vi "Loop_SEN.vi"() -> ()   [LabVIEW 2017, in "TemplateSensor.lvlib"]
uses:
  TemplateSensor.lvlib
  _SHARE ALL/Global Share All/Global_STOP.vi
  Global_CMD.vi
  Global_SEN Write_Data.vi
panel:
  out "Output Data":dbl
  out "Input Data":bool
  out "Cycle Time (S)":dbl format="%.3g"
  in  "Target Time(ms)":u32=50
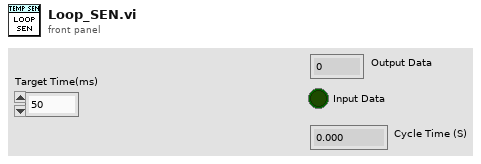
[diagram p1: front panel]
types:
  T1 = cluster{"Sensor Ref Data":cluster{i32}, " Sensor Output":dbl, "Sesnor Input":bool, "Target Time(ms)":u32, "Current Time":timestamp, "Previous Time":timestamp, "Cycle Time (S)":dbl}
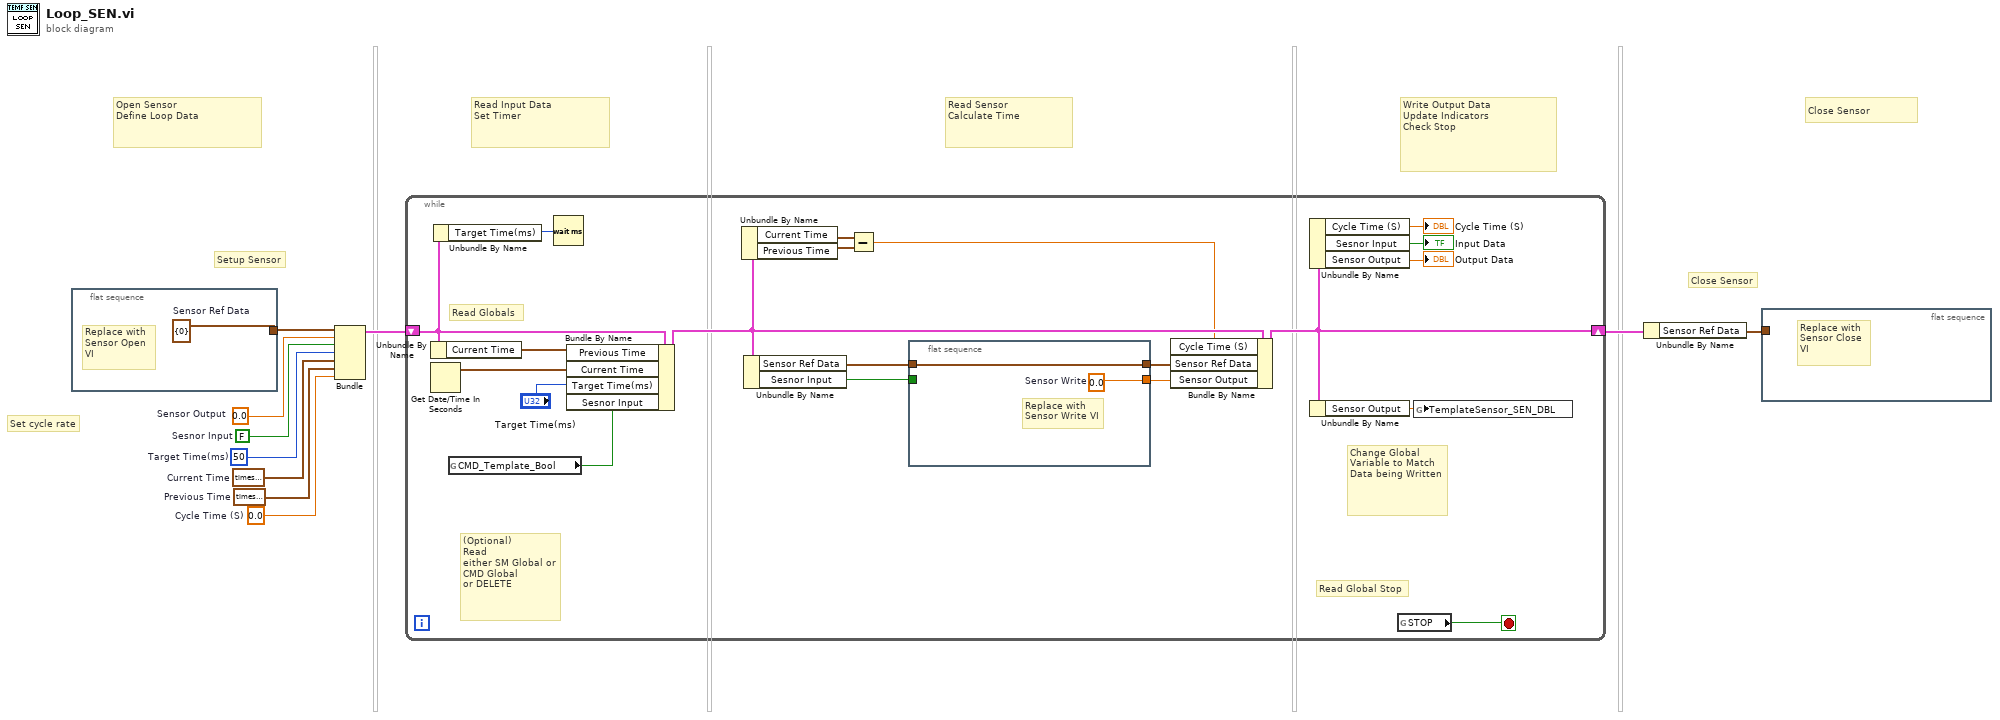
[diagram p0: block diagram]
diagram:
  w1 = 0.0  # Cycle Time (S)
  w10 = timestamp(0 s since 1904-01-01)  # Previous Time
  w9 = timestamp(0 s since 1904-01-01)  # Current Time
  w8 = u32 50  # Target Time(ms)
  w6 = FALSE  # Sesnor Input
  w4 = 0.0  # Sensor Output
  # "Close Sensor"
  # "Write Output Data\nUpdate Indicators\nCheck Stop"
  # "Read Sensor\nCalculate Time"
  # "Read Input Data\nSet Timer"
  # "Open Sensor\nDefine Loop Data"
  # "Set cycle rate"
  # "Close Sensor"
  # "Setup Sensor"
  n1 = flat-sequence {
    tunnel: [w11] -> w3
    frame #0 {
      w11 = cluster{i32} {0}  # Sensor Ref Data
      # "Replace with \nSensor Open\nVI"
    }
  }
  n2 = Bundle("Sensor Ref Data"=w3, "Sensor Output"=w4, "Sesnor Input"=w6, "Target Time(ms)"=w8, "Current Time"=w9, "Previous Time"=w10, "Cycle Time (S)"=w1) -> (w5:T1)  [unwired: 1 in]
  n3 = while {
    shift-right: [w17] -> w2
    shift-left: w5 -> [w19]
    stop <- w31 stop-if-true
    # "Change Global\nVariable to Match\nData being Written"
    # "(Optional)\nRead\neither SM Global or CMD Global\nor DELETE"
    # "Read Globals"
    # "Read Global Stop"
    n4 = Unbundle By Name(w19) -> ("Current Time"=w24:timestamp)
    n5 = Get Date/Time In Seconds() -> (seconds since 1Jan1904=w25:timestamp)
    n6 = Unbundle By Name(w19) -> ("Target Time(ms)"=w18:u32)
    n7 = global read "Global_CMD.vi" "CMD_Template_Bool"() -> (w12:bool)
    n8 = Wait (ms)(milliseconds to wait=w18) -> ()  [unwired: 1 out]
    n9 = Bundle By Name(cluster=w19, "Previous Time"=w24, "Current Time"=w25, "Target Time(ms)"="Target Time(ms)", "Sesnor Input"=w12) -> (w20:T1)
    n10 = Unbundle By Name(w20) -> ("Current Time"=w23:timestamp, "Previous Time"=w22:timestamp)
    n11 = Unbundle By Name(w20) -> ("Sensor Ref Data"=w30:cluster{i32}, "Sesnor Input"=w27:bool)
    n12 = Subtract(x=w23, y=w22) -> (x-y=w13:dbl)
    n13 = flat-sequence {
      tunnel: w30 -> [w33]
      tunnel: [w33] -> w29
      tunnel: [w32] -> w26
      tunnel: w27 -> [_]
      frame #0 {
        w32 = 0.0  # Sensor Write
        # "Replace with\nSensor Write VI"
      }
    }
    n14 = Bundle By Name(cluster=w20, "Cycle Time (S)"=w13, "Sensor Ref Data"=w29, "Sensor Output"=w26) -> (w17:T1)
    n15 = Unbundle By Name(w17) -> ("Cycle Time (S)"=→"Cycle Time (S)":dbl, "Sesnor Input"=→"Input Data":bool, "Sensor Output"=→"Output Data":dbl)
    n16 = Unbundle By Name(w17) -> ("Sensor Output"=w28:dbl)
    n17 = global read "Global_STOP.vi" "STOP"() -> (w31:bool)
    n18 = global write "Global_SEN Write_Data.vi" "TemplateSensor_SEN_DBL"(w28) -> ()
  }
  n19 = Unbundle By Name(w2) -> ("Sensor Ref Data"=w7:cluster{i32})
  n20 = flat-sequence {
    tunnel: w7 -> [_]
    frame #0 {
      # "Replace with \nSensor Close\nVI"
    }
  }
